vi "Draw Color Frame.vi"(8 "error in (no error)":errorcluster, 10 "Byte Array":u8[](array[numeric]), 11 "Image":T1) -> (0 "error out":errorcluster, 3 "Image Out":T1)   [LabVIEW 2014]
uses:
  <vilib>/vision/Image Controls.llb/IMAQ Image.ctl
  Frame Description FGV [Color].vi
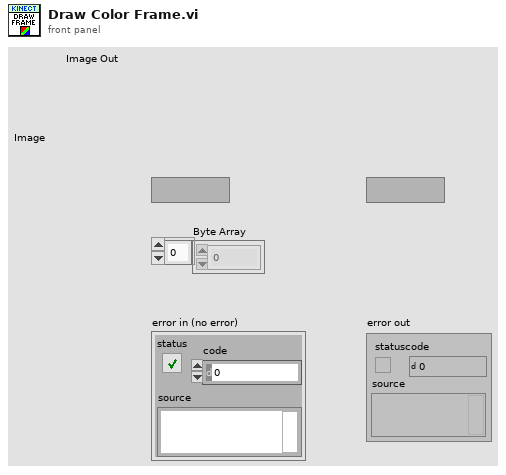
[diagram p1: front panel]
types:
  T1 = typedef "IMAQ Image.ctl" = refnum<image>
  T2 = typedef "FrameDescription.ctl" = cluster{"BytesPerPixel":u32, "DiagonalFieldOfView":sgl, "Height":i32, "HorizontalFieldOfView":sgl, "LengthInPixels":u32, "VerticalFieldOfView":sgl, "Width":i32}
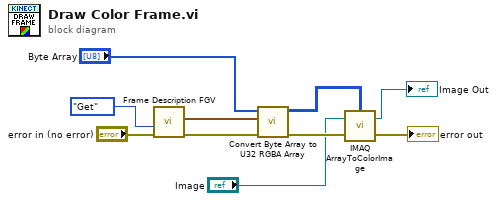
[diagram p0: block diagram]
diagram:
  n1 = call-poly "Frame Description FGV.vi"("error in (no error)"="error in (no error)", "Command"=enum16{"Get", "Set"}."Get") -> ("error out"=w3:errorcluster, "FrameDescription"=w2:T2)  [unwired: 8 in]
  n2 = call "Convert Byte Array to U32 RGBA Array.vi"("error in (no error)"=w3, "FrameDescription"=w2, "Byte Array"="Byte Array") -> ("error out"=w10:errorcluster, "RGBA U32 Array"=w9:u32[][])  [unwired: 7 in]
  n3 = call "IMAQ ArrayToColorImage"("Image Pixels (U32)"=w9, "Image"="Image", "error in (no error)"=w10) -> ("Image Out"=→"Image Out":T1, "error out"=→"error out":errorcluster)  [unwired: 2 in]
